vi "fg_Functional parameters.vi"(9 "Function":T6, 11 "Functional Parameters in":T5={"ROI data"=[], "ROI format version"=-1, "Norm ROI data"=[], "Norm. ROI format version"=-1, "Z norm"=[], "Z norm format version"=-1}) -> (0 "[ROI vis]":T1 {"ROI number" min=1 format="ROI %.0f"}, 1 "ROI indexes by type":T4, 2 "# of ROI":i32, 3 "Functional Parameters":T5={"ROI data"=[], "ROI format version"=-1, "Norm ROI data"=[], "Norm. ROI format version"=-1, "Z norm"=[], "Z norm format version"=-1})   [LabVIEW 2013]
uses:
  Typedefs/Get-Set-Clear Control.ctl
  Typedefs/Functional Parameters Cluster.ctl
  Typedefs/ROI indexes by type.ctl
  Typedefs/ROI selector array-ROI vis.ctl
  xcontrol/Interface VIs/Interface typedefs/Interface-ROI selection cluster.ctl
  Typedefs/ROI ID Enum.ctl
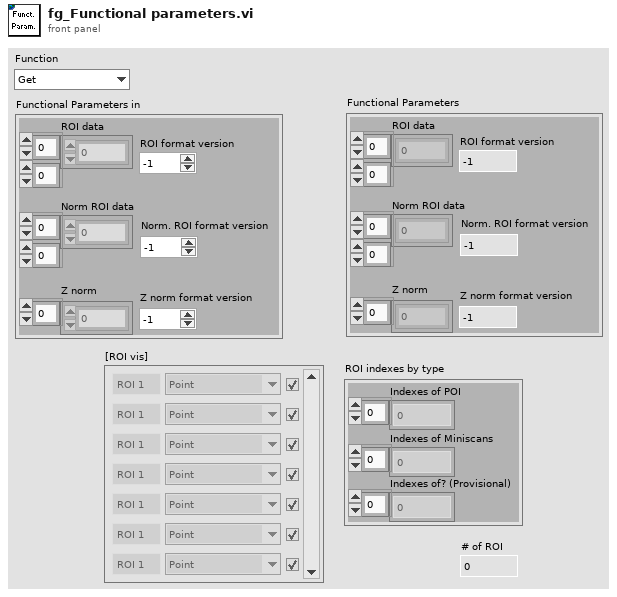
[diagram p1: front panel]
types:
  T1 = typedef "ROI selector array-ROI vis.ctl" = T2[]
  T2 = typedef "Interface-ROI selection cluster.ctl" = cluster{"ROI number":i32, "ROI ID":T3, "Visibility":bool}
  T3 = typedef "ROI ID Enum.ctl" = enum16{"Point", "MiniScan", "Comp. MiniScan", "Rectangle", "Comp. volume", "Arb. plane point"}
  T4 = typedef "ROI indexes by type.ctl" = cluster{"Indexes of POI":i32[], "Indexes of Miniscans":i32[], "Indexes of? (Provisional)":i32[]}
  T5 = typedef "Functional Parameters Cluster.ctl" = cluster{"ROI data":dbl[][], "ROI format version":i32, "Norm ROI data":dbl[][], "Norm. ROI format version":i32, "Z norm":dbl[], "Z norm format version":i32}
  T6 = typedef "Get-Set-Clear Control.ctl" = enum16{"Get", "Set", "Clear"}
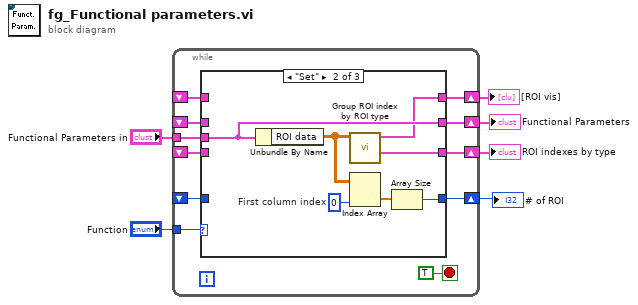
[diagram p0: block diagram]
diagram:
  n1 = while {
    shift-right: [w16] -> w4
    shift-left: _ -> [w14]
    tunnel: "Functional Parameters in" -> [w15]
    tunnel: "Function" -> [w13]
    shift-right: [w12] -> w3
    shift-left: _ -> [w11]
    shift-right: [w10] -> w2
    shift-left: _ -> [w9]
    shift-right: [w8] -> w1
    shift-left: _ -> [w7]
    stop <- TRUE stop-if-true
    n2 = case shown="\"Set\"" w13 {
      tunnel: [w21 w28 _] -> w16
      tunnel: w15 -> [_ w28 _]
      tunnel: w14 -> [w21 _ _]
      tunnel: [w20 w27 _] -> w12
      tunnel: w11 -> [w20 _ _]
      tunnel: [w19 w23 _] -> w10
      tunnel: w9 -> [w19 _ _]
      tunnel: [w18 w22 _] -> w8
      tunnel: w7 -> [w18 _ _]
      frame "Get", Default {
      }
      frame "Set" {
        w25 = 0  # First column index
        n3 = Unbundle By Name(w28) -> ("ROI data"=w24:dbl[][])
        n4 = call "Group ROI index by ROI type.vi"("ROI data"=w24) -> ("ROI indexes by type"=w27:T4, "[ROI vis]"=w22:T1)  [unwired: 9 in]
        n5 = Index Array(array=w24, index (col)=w25) -> (element=w26:dbl[])  [unwired: 1 in]
        n6 = Array Size(array=w26) -> (size(s)=w23:i32)
      }
      frame "Clear" {
      }
    }
  }
  "Functional Parameters" <- w4
  "ROI indexes by type" <- w3
  "# of ROI" <- w2
  "[ROI vis]" <- w1
